vi "Host3.vi"() -> ()   [LabVIEW 2025]
uses:
  <vilib>/numeric/Random Number (Range) U64.vi
  <vilib>/Analysis/baseanly.llb/Real Dot Product.vi
  <vilib>/Analysis/baseanly.llb/Real A x B.vi
  <vilib>/numeric/sub_Random U32.vi
  <vilib>/Analysis/Matrix/Numeric/Conversions/Matrix To Array - RM.vi
  <vilib>/FPGAPlugInAG/cRIO-9033/niLvFpga_Open_cRIO-9033.vi
  <vilib>/rvi/interface/common/dynamic/niFpgaDynamicAddResources.vi
  <vilib>/FPGAPlugInAG/Dynamic/niLvFpga_Reset_Dynamic.vi
  <vilib>/FPGAPlugInAG/Dynamic/niLvFpga_Run_Dynamic.vi
  <vilib>/Utility/error.llb/Error Cluster From Error Code.vi
  <vilib>/rvi/errors/niLvFpgaAdjustHostInterfaceError.vi
  <vilib>/FPGAPlugInAG/Dynamic/niLvFpga_Close_Dynamic.vi
  <vilib>/rvi/interface/nirviOpenFPGA/nirviOpenFPGA.xnode
  FPGA Bitfiles/dotplot9033_FPGATarget_Target3_4TiCGxcWVlU.lvbitx
  <vilib>/rvi/interface/nirviMethod/nirviMethod.xnode
  <vilib>/rvi/interface/nirviReadWriteControl/nirviReadWriteControl.xnode
  <vilib>/rvi/interface/nirviCloseFPGA/nirviCloseFPGA.xnode
  <vilib>/Analysis/NI_AALBase.lvlib
  <vilib>/Analysis/Matrix/NI_Matrix.lvlib
  <vilib>/FPGAPlugInAG/Dynamic/niLvFpga_ReadFifo_Dynamic.vi
  <vilib>/rvi/errors/niLvFpgaMergeErrorWithErrorCode.vi
  NiFpgaLv.dll
  <vilib>/rvi/interface/Simulation/niFpgaSimulationCallBeginRW.vi
panel:
  out "Numeric":i32
  out "cr":fxp<+/-,32,16>[](array[numeric])
  out "Data":fxp<+/-,32,16>[](array[numeric])
  out "Elements Remaining":u32
  out "FIFO A Input":fxp<+/-,32,16>[](array[numeric])
  out "FIFO B Input":fxp<+/-,32,16>[](array[numeric])
  out "X * Y":fxp<+/-,64,32>
  out "elements in B":i32
  out "elements in A":i32
  out "elements in C":i32
  out "C - Real":dbl[][](array[numeric])
  out "B":fxp<+/-,32,16>[][](array[numeric])
  out "A":fxp<+/-,32,16>[][](array[numeric])
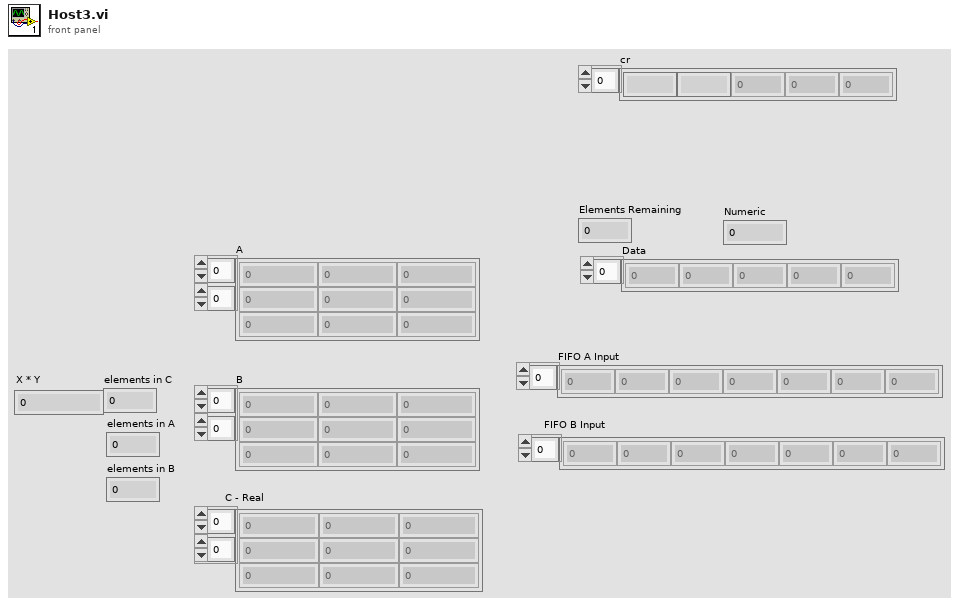
[diagram p1: front panel]
types:
  T1 = typedef "NI_Matrix.lvlib/RealMatrix.ctl" = dbl[][]
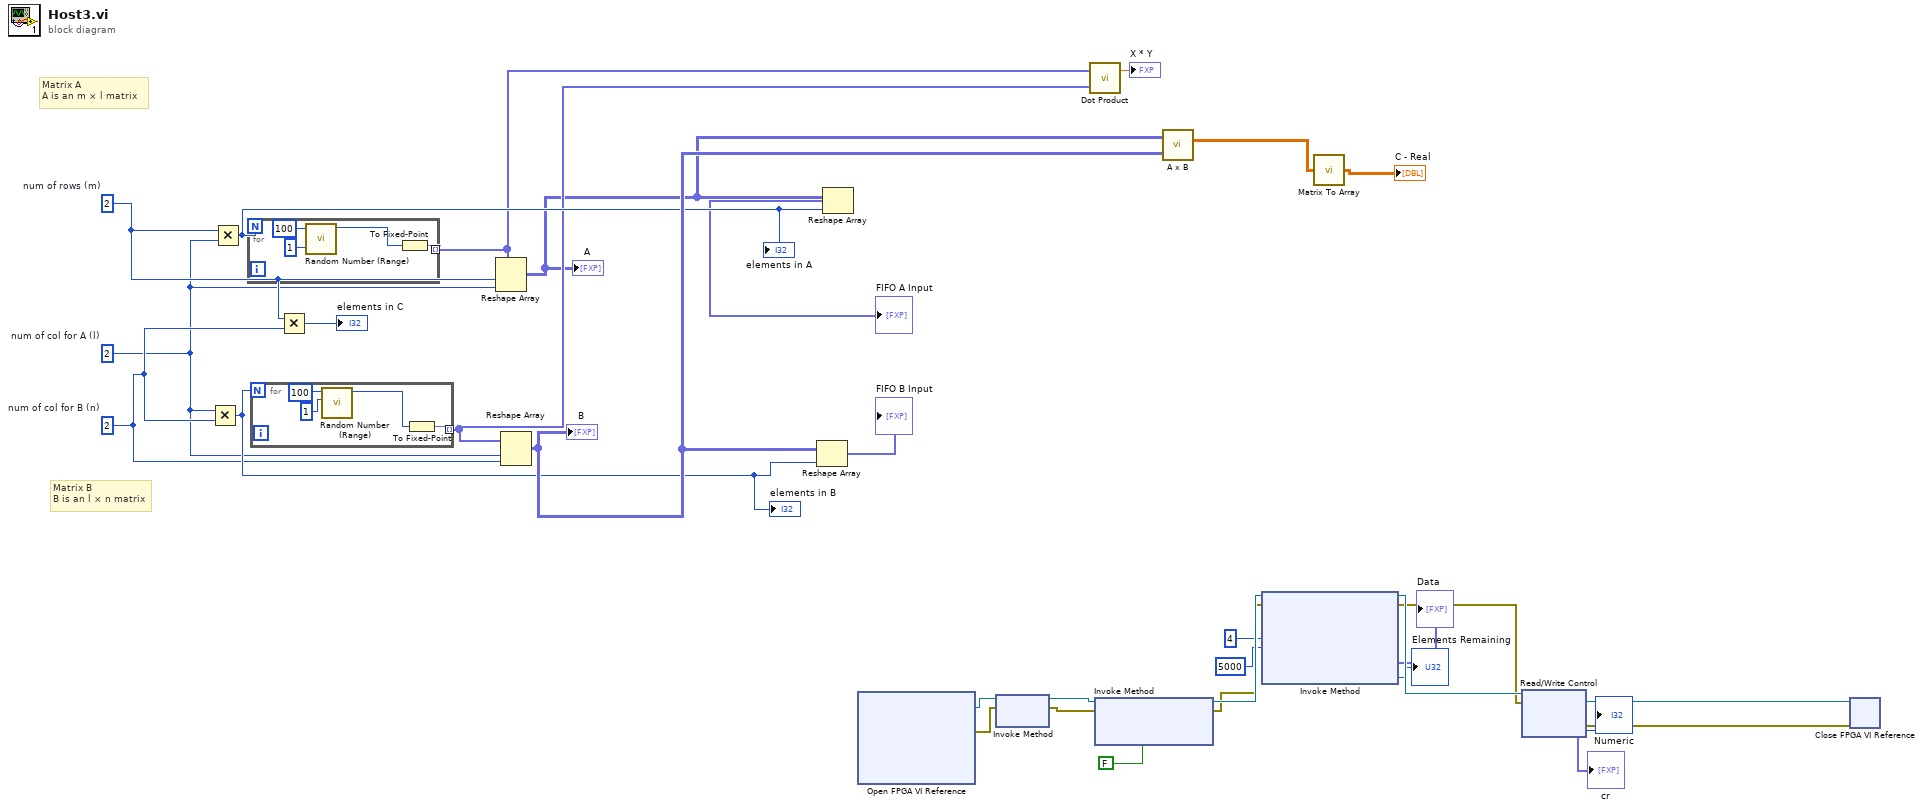
[diagram p0: block diagram]
diagram:
  w21 = 2  # num of col for B (n)
  w20 = 2  # num of col for A (l)
  w28 = 2  # num of rows (m)
  # "Matrix B\nB is an l × n matrix"
  # "Matrix A\nA is an m × l matrix"
  n1 = Multiply(x=w20, y=w21) -> (x*y=w26:i32)
  "elements in B" <- w26
  n2 = Multiply(x=w28, y=w20) -> (x*y=w30:i32)
  "elements in A" <- w30
  n3 = for {
    N: w30 -> [_]
    tunnel: [w36] -> w25 mode=indexing
    n4 = call-poly <vilib>:"Random Number (Range).vi"("lower bound (0)"=u64 1, "upper bound (100)"=u64 100) -> ("number"=w35:u64)  [unwired: 9 in]
    n5 = To Fixed-Point(number=w35) -> (fixed-point=w36:fxp<+,64,64>)  [unwired: 1 in]
  }
  n6 = for {
    N: w26 -> [_]
    tunnel: [w40] -> w24 mode=indexing
    n7 = call-poly <vilib>:"Random Number (Range).vi"("lower bound (0)"=u64 1, "upper bound (100)"=u64 100) -> ("number"=w37:u64)  [unwired: 9 in]
    n8 = To Fixed-Point(number=w37) -> (fixed-point=w40:fxp<+,64,64>)  [unwired: 1 in]
  }
  n9 = Multiply(x=w28, y=w21) -> (x*y=→"elements in C":i32)
  n10 = Reshape Array(w25, w28, w20) -> (w22:fxp<+,64,64>[][])
  "A" <- w22
  n11 = Reshape Array(w24, w20, w21) -> (w32:fxp<+,64,64>[][])
  "B" <- w32
  n12 = Reshape Array(w32, w26) -> (→"FIFO B Input":fxp<+,64,64>[])
  n13 = Reshape Array(w22, w30) -> (→"FIFO A Input":fxp<+,64,64>[])
  n14 = xnode "Open FPGA VI Reference"() -> ("FPGA VI Reference Out"=w18:refnum<k20>, "error out"=w17:errorcluster)  [unwired: 2 in]
  n15 = xnode "Invoke Method"("FPGA VI Reference In"=w18, "error in"=w17) -> ("FPGA VI Reference Out"=w14:refnum<k20>, "error out"=w15:errorcluster)
  n16 = call-poly <vilib>:"Dot Product.vi"("Y Vector"=w24, "X Vector"=w25) -> ("X * Y"=→"X * Y":dbl)  [unwired: 1 out]
  n17 = xnode "Invoke Method"("FPGA VI Reference In"=w14, "error in"=w15, "Wait Until Done (F)"=FALSE) -> ("FPGA VI Reference Out"=w11:refnum<k20>, "error out"=w10:errorcluster)
  n18 = call-poly <vilib>:"A x B.vi"("B"=w32, "A"=w22) -> ("A x B"=w31:T1)  [unwired: 1 out]
  n19 = xnode "Invoke Method"("FPGA VI Reference In"=w11, "error in"=w10, "Number of Elements"=u32 4, "Timeout (ms)"=5000) -> ("FPGA VI Reference Out"=w8:refnum<k20>, "error out"=w7:errorcluster, "Data"=→"Data":fxp<+/-,32,16>[], "Elements Remaining"=→"Elements Remaining":u32)
  n20 = call-poly <vilib>:"Matrix To Array.vi"("Real Matrix"=w31) -> ("Real 2D Array"=→"C - Real":dbl[][])
  n21 = xnode "Read/Write Control"("FPGA VI Reference In"=w8, "error in"=w7) -> ("FPGA VI Reference Out"=w13:refnum<k20>, "error out"=w12:errorcluster, "cr"=→"cr":fxp<+/-,32,16>[], "Numeric"=→"Numeric":i32)
  n22 = xnode "Close FPGA VI Reference"("FPGA VI Reference In"=w13, "error in"=w12) -> ()  [unwired: 1 out]
